vi "GetType.vi"(8 "error in (no error)":errorcluster, 11 "Clear Arbitrary Memory [SEQ] Msg in":refnum<class "Clear Arbitrary Memory [SEQ] Msg.lvclass">) -> (0 "error out":errorcluster, 2 "Data Sample":variant, 3 "Clear Arbitrary Memory [SEQ] Msg out":refnum<class "Clear Arbitrary Memory [SEQ] Msg.lvclass">)   [LabVIEW 2014, in "CS++Fgen.lvlib" / "Clear Arbitrary Memory [SEQ] Msg.lvclass"]
doc: "This VI delivers a sample of the data type format the message expects."
uses:
  Clear Arbitrary Memory [SEQ] Msg.lvclass
  Clear Arbitrary Memory [SEQ] Msg.lvclass/Clear Arbitrary Memory [SEQ] Msg.ctl
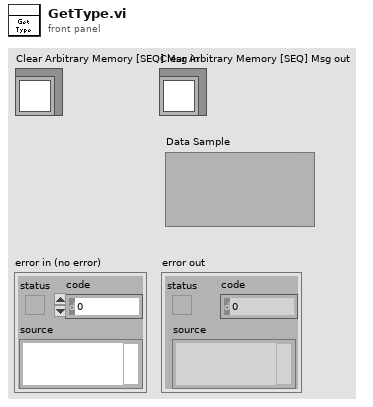
[diagram p1: front panel]
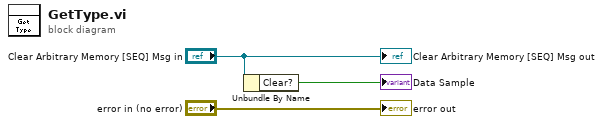
[diagram p0: block diagram]
diagram:
  n1 = Unbundle By Name("Clear Arbitrary Memory [SEQ] Msg in") -> ("Clear?"=→"Data Sample":bool)
  "error out" <- "error in (no error)"
  "Clear Arbitrary Memory [SEQ] Msg out" <- "Clear Arbitrary Memory [SEQ] Msg in"
